vi "Teleop.vi"(10 "Match Info":T1={"Autonomous Elapsed Seconds"=0.0, "TeleOp Elapsed Seconds"=0.0, "Disabled Elapsed Seconds"=0.0, "Visited Autonomous"=FALSE, "Visited TeleOp"=FALSE, "Visited Disabled"=FALSE, "Autonomous Settings"={"Autonomous Style"=enum."Independent", "VI Refnum"=refnum}}, 11 "Call Context":T2) -> ()   [LabVIEW 2019]
doc: "This VI is called for each TeleOp packet received from the DS where the robot is not disabled. It is often used to read from the joysticks and update I/O or to update setpoints for timed control loops. It should complete and return within 20 milliseconds or it may miss DS packets."
uses:
  <vilib>/Rock Robotics/Network Tables/NT Write Numeric Array.vi
  Robot Global Data.vi
  <vilib>/Rock Robotics/Network Tables/NT Write Number.vi
  <vilib>/Rock Robotics/Network Tables/NT Write Boolean.vi
  <vilib>/Rock Robotics/Network Tables/NT Write Boolean Array.vi
  <vilib>/Rock Robotics/WPI/DriverStation/WPI_DriverStationMatch Info.ctl
  <vilib>/Rock Robotics/WPI/DriverStation/WPI_DriverStationDerivedRobotMode.ctl
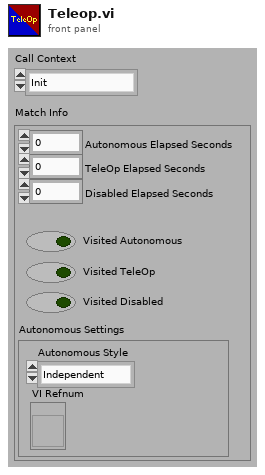
[diagram p1: front panel]
types:
  T1 = typedef "WPI_DriverStationMatch Info.ctl" = cluster{"Autonomous Elapsed Seconds":dbl, "TeleOp Elapsed Seconds":dbl, "Disabled Elapsed Seconds":dbl, "Visited Autonomous":bool, "Visited TeleOp":bool, "Visited Disabled":bool, "Autonomous Settings":cluster{"Autonomous Style":enum16{"Iterative", "Independent"}, "VI Refnum":refnum<vi>}}
  T2 = typedef "WPI_DriverStationDerivedRobotMode.ctl" = enum16{"Init", "Execute", "Stop"}
  T3 = typedef "WPI_JoystickDevRef.ctl" = cluster{"Device":T4}
  T4 = typedef "WPI_JoystickDeviceEnum.ctl" = enum16{"USB 0", "USB 1", "USB 2", "USB 3", "USB 4", "USB 5"}
  T5 = typedef "WPI_RobotDriveDevRef.ctl" = cluster{"DevStatus":errorcluster, "Motors[]":T6[], "Square Inputs":bool, "Max Output":dbl}
  T6 = typedef "WPI_MotorControlDeviceRef.ctl" = cluster{"DeviceStatus":errorcluster, "Type":T7, "PWM":cluster{"PWM Channel":T8, "DeadBand":T9}, "CAN":cluster{"Device Number":u8, "SetOutput VI Ref":variant, "GetOutput VI Ref":variant, "Enable VI Ref":variant, "Disable VI Ref":variant, "Data":variant}, "Invert":bool, "DIO PWM":cluster{"PWM \"Enable\" Channel":T8, "DIOChannel":T10, "PWM Rate":dbl}}
  T7 = typedef "WPI_MotorControlType.ctl" = enum16{"PWM", "CAN", "DIO PWM"}
  T8 = typedef "FPGA_DIOPWMChannel.ctl" = enum8{"PWM 0", "PWM 1", "PWM 2", "PWM 3", "PWM 4", "PWM 5", "PWM 6", "PWM 7", "PWM 8", "PWM 9", "PWM MXP 0", "PWM MXP 1", "PWM MXP 2", "PWM MXP 3", "PWM MXP 4", "PWM MXP 5", "PWM MXP 6", "PWM MXP 7", "PWM MXP 8", "PWM MXP 9", "Invalid"}
  T9 = typedef "WPI_PWMDeadband.ctl" = cluster{"Name":string, "maxPositivePwm":i32, "minPositivePwm":i32, "centerPwm":i32, "maxNegativePwm":i32, "minNegativePwm":i32, "angularRange":u16}
  T10 = typedef "FPGA_DIOChannel.ctl" = enum8{"DIO 0", "DIO 1", "DIO 2", "DIO 3", "DIO 4", "DIO 5", "DIO 6", "DIO 7", "DIO 8", "DIO 9", "DIO MXP 0", "DIO MXP 1", "DIO MXP 2", "DIO MXP 3", "DIO MXP 4", "DIO MXP 5", "DIO MXP 6", "DIO MXP 7", "DIO MXP 8", "DIO MXP 9", "DIO MXP 10", "DIO MXP 11", "DIO MXP 12", "DIO MXP 13", "DIO MXP 14", "DIO MXP 15", "SPI Port CS1", "SPI Port CS2", "SPI Port CS3", "SPI Port MISO", "SPI Port MOSI", "Invalid"}
  T11 = typedef "WPI_SwitchDevRef.ctl" = cluster{"DevStatus":errorcluster, "DIO Channel":T10, "CntIndex":T12, "Normally Closed":bool}
  T12 = typedef "FPGA_CounterCtrSystemIndex.ctl" = enum8{"Ctr 0", "Ctr 1", "Ctr 2", "Ctr 3", "Ctr 4", "Ctr 5", "Ctr 6", "Ctr 7", "Invalid"}
  T13 = cluster{"JoystickDevRef":T3, "RobotDriveDevRef":T5}
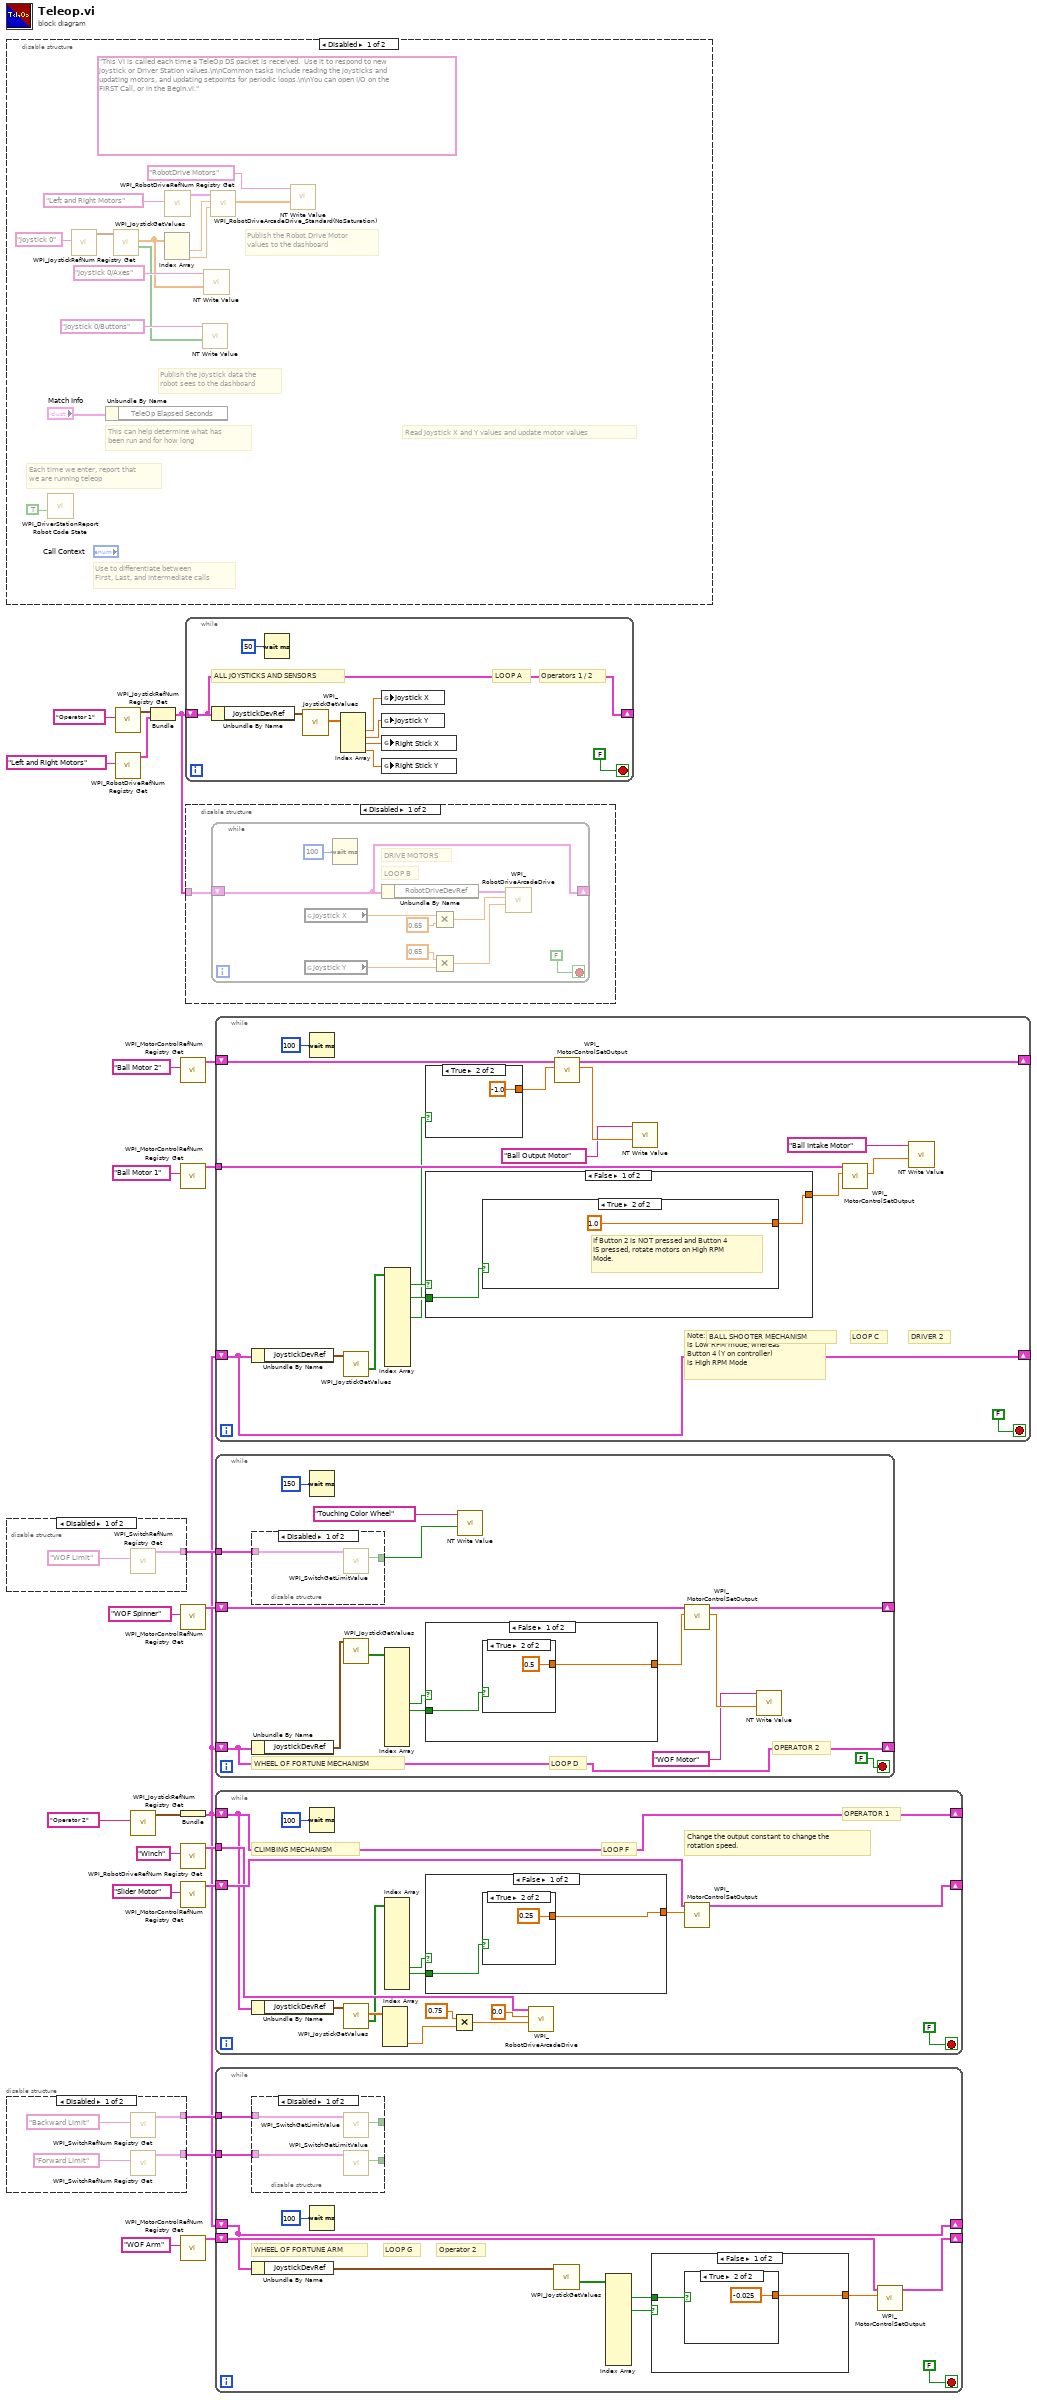
[diagram p0: block diagram]
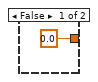
[diagram p4: hidden frame]
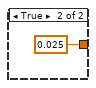
[diagram p5: hidden frame]
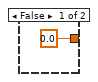
[diagram p7: hidden frame]
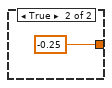
[diagram p8: hidden frame]
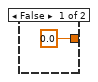
[diagram p12: hidden frame]
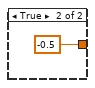
[diagram p13: hidden frame]
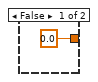
[diagram p14: hidden frame]
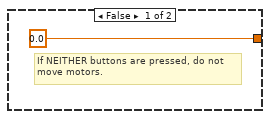
[diagram p15: hidden frame]
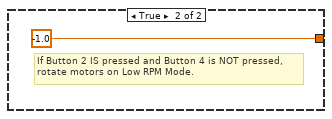
[diagram p16: hidden frame]
diagram:
  n1 = disable-structure shown="Disabled" {
    frame Disabled {
      (unwired) "This VI is called each time a TeleOp DS packet is received.  Use it to respond to new joystick or Driver Station values.\n\nCommon tasks include reading the joysticks and updating motors, and updating setpoints for periodic loops.\n\nYou can open I/O on the FIRST Call, or in the Begin.vi."
      # "Publish the Robot Drive Motor\nvalues to the dashboard"
      # "Publish the joystick data the\nrobot sees to the dashboard"
      # "Each time we enter, report that\nwe are running teleop"
      # "Use to differentiate between\nFirst, Last, and Intermediate calls"
      # "This can help determine what has\nbeen run and for how long"
      # "Read Joystick X and Y values and update motor values"
      n2 = call <vilib>:"WPI_DriverStationReport Robot Code State.vi"("TeleOp"=TRUE ("Autonomous")) -> ()  [unwired: 10 in, 1 out]
      n3 = call <vilib>:"WPI_JoystickRefNum Registry Get.vi"("refnum name"="Joystick 0") -> ("JoystickDevRef"=w32:T3)  [unwired: 1 in, 9 out]
      n4 = Unbundle By Name("Match Info") -> ()  [unwired: 1 out]
      n5 = call <vilib>:"WPI_JoystickGetValues.vi"("JoystickDevRef"=w32) -> ("Buttons"=w26:bool[], "Axes"=w27:dbl[])  [unwired: 6 in, 3 out]
      n6 = Index Array(array=w27) -> (element #1=w34:dbl, element #2=w30:dbl)  [unwired: 2 in]
      n7 = call <vilib>:"WPI_RobotDriveRefNum Registry Get.vi"("refnum name"="Left and Right Motors") -> ("RobotDriveDevRef"=w35:T5)  [unwired: 1 in, 9 out]
      n8 = call-poly <vilib>:"NT Write Value.vi"("Boolean Array"=w26, "Name"="Joystick 0/Buttons") -> ()  [unwired: 9 in, 1 out]
      n9 = call-poly <vilib>:"NT Write Value.vi"("Numeric Array"=w27, "Name"="Joystick 0/Axes") -> ()  [unwired: 9 in, 1 out]
      n10 = call <vilib>:"WPI_RobotDriveArcadeDrive_Standard(NoSaturation).vi"("Y axis value"=w30, "X axis value"=w34, "RobotDriveDevRef"=w35) -> ("Motor Values"=w25:dbl[])  [unwired: 1 in, 7 out]
      n11 = call-poly <vilib>:"NT Write Value.vi"("Numeric Array"=w25, "Name"="RobotDrive Motors") -> ()  [unwired: 9 in, 1 out]
    }
    frame Enabled {
    }
  }
  n12 = disable-structure shown="Disabled" {
    disable-tunnel: [w38 _] -> w13
    frame Disabled {
      n13 = call <vilib>:"WPI_SwitchRefNum Registry Get.vi"("refnum name"="WOF Limit") -> ("SwitchDevRef"=w38:T11)  [unwired: 9 in, 1 out]
    }
    frame Enabled {
    }
  }
  n14 = disable-structure shown="Disabled" {
    disable-tunnel: [w41 _] -> w8
    disable-tunnel: [w40 _] -> w7
    frame Disabled {
      n15 = call <vilib>:"WPI_SwitchRefNum Registry Get.vi"("refnum name"="Backward Limit") -> ("SwitchDevRef"=w40:T11)  [unwired: 9 in, 1 out]
      n16 = call <vilib>:"WPI_SwitchRefNum Registry Get.vi"("refnum name"="Forward Limit") -> ("SwitchDevRef"=w41:T11)  [unwired: 9 in, 1 out]
    }
    frame Enabled {
    }
  }
  n17 = call <vilib>:"WPI_JoystickRefNum Registry Get.vi"("refnum name"="Operator 1") -> ("JoystickDevRef"=w21:T3)  [unwired: 1 in, 9 out]
  n18 = call <vilib>:"WPI_RobotDriveRefNum Registry Get.vi"("refnum name"="Left and Right Motors") -> ("RobotDriveDevRef"=w20:T5)  [unwired: 1 in, 9 out]
  n19 = call <vilib>:"WPI_JoystickRefNum Registry Get.vi"("refnum name"="Operator 2") -> ("JoystickDevRef"=w5:T3)  [unwired: 9 in, 1 out]
  n20 = Bundle("JoystickDevRef"=w21, "RobotDriveDevRef"=w20) -> (w2:T13)  [unwired: 1 out]
  n21 = call <vilib>:"WPI_MotorControlRefNum Registry Get.vi"("refnum name"="Ball Motor 2") -> ("MotorControlDevRef"=w14:T6)  [unwired: 9 in, 1 out]
  n22 = call <vilib>:"WPI_MotorControlRefNum Registry Get.vi"("refnum name"="Ball Motor 1") -> ("MotorControlDevRef"=w18:T6)  [unwired: 9 in, 1 out]
  n23 = call <vilib>:"WPI_MotorControlRefNum Registry Get.vi"("refnum name"="WOF Spinner") -> ("MotorControlDevRef"=w16:T6)  [unwired: 9 in, 1 out]
  n24 = Bundle("JoystickDevRef"=w5) -> (w1:cluster{"JoystickDevRef":T3})  [unwired: 1 in]
  n25 = call <vilib>:"WPI_RobotDriveRefNum Registry Get.vi"("refnum name"="Winch") -> ("RobotDriveDevRef"=w4:T5)  [unwired: 9 in, 1 out]
  n26 = call <vilib>:"WPI_MotorControlRefNum Registry Get.vi"("refnum name"="Slider Motor") -> ("MotorControlDevRef"=w12:T6)  [unwired: 9 in, 1 out]
  n27 = call <vilib>:"WPI_MotorControlRefNum Registry Get.vi"("refnum name"="WOF Arm") -> ("MotorControlDevRef"=w10:T6)  [unwired: 9 in, 1 out]
  n28 = while {
    shift-right: [w51] -> _
    shift-left: w2 -> [w51]
    stop <- FALSE stop-if-true
    # "Operators 1 / 2"
    # "LOOP A"
    # "ALL JOYSTICKS AND SENSORS"
    n29 = Unbundle By Name(w51) -> ("JoystickDevRef"=w50:T3)
    n30 = Wait (ms)(milliseconds to wait=u32 50) -> ()  [unwired: 1 out]
    n31 = call <vilib>:"WPI_JoystickGetValues.vi"("JoystickDevRef"=w50) -> ("Axes"=w49:dbl[])  [unwired: 6 in, 4 out]
    n32 = Index Array(array=w49) -> (element #1=w47:dbl, element #2=w48:dbl, element #3=w45:dbl, element #4=w44:dbl)  [unwired: 4 in]
    n33 = global write "Robot Global Data.vi" "Joystick X"(w47) -> ()
    n34 = global write "Robot Global Data.vi" "Joystick Y"(w48) -> ()
    n35 = global write "Robot Global Data.vi" "Right Stick X"(w45) -> ()
    n36 = global write "Robot Global Data.vi" "Right Stick Y"(w44) -> ()
  }
  n37 = disable-structure shown="Disabled" {
    disable-tunnel: w2 -> [w53 _]
    frame Disabled {
      n38 = while {
        shift-right: [w61] -> _
        shift-left: w53 -> [w61]
        stop <- FALSE stop-if-true
        # "DRIVE MOTORS"
        # "LOOP B"
        n39 = global read "Robot Global Data.vi" "Joystick X"() -> (w58:dbl)
        n40 = global read "Robot Global Data.vi" "Joystick Y"() -> (w59:dbl)
        n41 = Wait (ms)(milliseconds to wait=u32 100) -> ()  [unwired: 1 out]
        n42 = Unbundle By Name(w61) -> ("RobotDriveDevRef"=w60:T5)
        n43 = Multiply(x=w58, y=0.65) -> (x*y=w54:dbl)
        n44 = Multiply(x=0.65, y=w59) -> (x*y=w55:dbl)
        n45 = call-poly <vilib>:"WPI_RobotDriveArcadeDrive.vi"("Y axis value"=w55, "X axis value"=w54, "RobotDriveDevRef"=w60) -> ()  [unwired: 6 in, 3 out]
      }
    }
    frame Enabled {
    }
  }
  n46 = while {
    tunnel: w18 -> [w78]
    shift-right: [w74] -> _
    shift-left: w14 -> [w75]
    shift-right: [w65] -> _
    shift-left: w1 -> [w65]
    stop <- FALSE stop-if-true
    # "DRIVER 2"
    # "LOOP C"
    # "Note: Button 2 (A on controller) \nis Low RPM mode, whereas \nButton 4 (Y on controller)\nis High RPM Mode"
    # "BALL SHOOTER MECHANISM"
    n47 = Unbundle By Name(w65) -> ("JoystickDevRef"=w64:T3)
    n48 = Wait (ms)(milliseconds to wait=u32 100) -> ()  [unwired: 1 out]
    n49 = call <vilib>:"WPI_JoystickGetValues.vi"("JoystickDevRef"=w64) -> ("Buttons"=w76:bool[])  [unwired: 6 in, 4 out]
    n50 = Index Array(array=w76) -> (element #1=w73:bool, element #3=w72:bool, element #6=w70:bool)  [unwired: 13 in, 10 out]
    n51 = case shown="True" w70 {
      tunnel: [0.0 ("Output") -1.0 ("Output")] -> w71
      frame False {
      }
      frame True {
      }
    }
    n52 = case shown="False" w73 {
      tunnel: [w84 -1.0 ("Output")] -> w77
      tunnel: w72 -> [w83 _]
      frame False {
        n53 = case shown="True" w83 {
          tunnel: [0.0 ("Output") 1.0 ("Output")] -> w84
          frame False {
            # "If NEITHER buttons are pressed, do not\nmove motors."
          }
          frame True {
            # "If Button 2 is NOT pressed and Button 4\nIS pressed, rotate motors on High RPM\nMode."
          }
        }
      }
      frame True {
        # "If Button 2 IS pressed and Button 4 is NOT pressed,\nrotate motors on Low RPM Mode."
      }
    }
    n54 = call <vilib>:"WPI_MotorControlSetOutput.vi"("Output"=w71, "MotorControlDevRef"=w75) -> ("Motor Output"=w67:dbl, "MotorControlDevRef"=w74:T6)  [unwired: 7 in, 1 out]
    n55 = call-poly <vilib>:"NT Write Value.vi"("Numeric"=w67, "Name"="Ball Output Motor") -> ()  [unwired: 9 in, 1 out]
    n56 = call <vilib>:"WPI_MotorControlSetOutput.vi"("Output"=w77, "MotorControlDevRef"=w78) -> ("Motor Output"=w69:dbl)  [unwired: 7 in, 2 out]
    n57 = call-poly <vilib>:"NT Write Value.vi"("Numeric"=w69, "Name"="Ball Intake Motor") -> ()  [unwired: 9 in, 1 out]
  }
  n58 = while {
    shift-right: [w100] -> _
    shift-left: w16 -> [w101]
    tunnel: w13 -> [w97]
    shift-right: [w89] -> _
    shift-left: w1 -> [w89]
    stop <- FALSE stop-if-true
    # "OPERATOR 2"
    # "LOOP D"
    # "WHEEL OF FORTUNE MECHANISM"
    n59 = disable-structure shown="Disabled" {
      disable-tunnel: w97 -> [w104 _]
      disable-tunnel: [w103 _] -> w95
      frame Disabled {
        n60 = call <vilib>:"WPI_SwitchGetLimitValue.vi"("SwitchDevRef"=w104) -> ("Switch Pressed"=w103:bool)  [unwired: 8 in, 2 out]
      }
      frame Enabled {
      }
    }
    n61 = Unbundle By Name(w89) -> ("JoystickDevRef"=w88:T3)
    n62 = Wait (ms)(milliseconds to wait=u32 150) -> ()  [unwired: 1 out]
    n63 = call <vilib>:"WPI_JoystickGetValues.vi"("JoystickDevRef"=w88) -> ("Buttons"=w94:bool[])  [unwired: 6 in, 4 out]
    n64 = Index Array(array=w94) -> (element #7=w93:bool, element #8=w92:bool)  [unwired: 13 in, 11 out]
    n65 = case shown="False" w93 {
      tunnel: [w106 -0.5 ("Output")] -> w99
      tunnel: w92 -> [w105 _]
      frame False {
        n66 = case shown="True" w105 {
          tunnel: [0.0 ("Output") 0.5 ("Output")] -> w106
          frame False {
          }
          frame True {
          }
        }
      }
      frame True {
      }
    }
    n67 = call-poly <vilib>:"NT Write Value.vi"("Boolean"=w95, "Name"="Touching Color Wheel") -> ()  [unwired: 9 in, 1 out]
    n68 = call <vilib>:"WPI_MotorControlSetOutput.vi"("Output"=w99, "MotorControlDevRef"=w101) -> ("Motor Output"=w91:dbl, "MotorControlDevRef"=w100:T6)  [unwired: 7 in, 1 out]
    n69 = call-poly <vilib>:"NT Write Value.vi"("Numeric"=w91, "Name"="WOF Motor") -> ()  [unwired: 9 in, 1 out]
  }
  n70 = while {
    shift-right: [w110] -> _
    shift-left: w12 -> [w125]
    tunnel: w4 -> [w120]
    shift-right: [w112] -> _
    shift-left: w1 -> [w112]
    stop <- FALSE stop-if-true
    # "Change the output constant to change the\nrotation speed."
    # "OPERATOR 1"
    # "LOOP F"
    # "CLIMBING MECHANISM"
    n71 = Unbundle By Name(w112) -> ("JoystickDevRef"=w111:T3)
    n72 = Wait (ms)(milliseconds to wait=u32 100) -> ()  [unwired: 1 out]
    n73 = call <vilib>:"WPI_JoystickGetValues.vi"("JoystickDevRef"=w111) -> ("Buttons"=w115:bool[], "Axes"=w121:dbl[])  [unwired: 6 in, 3 out]
    n74 = Index Array(array=w121) -> (element #4=w117:dbl)  [unwired: 4 in, 3 out]
    n75 = Index Array(array=w115) -> (element #9=w114:bool, element #10=w113:bool)  [unwired: 12 in, 10 out]
    n76 = case shown="False" w114 {
      tunnel: [w127 -0.25 ("Output")] -> w123
      tunnel: w113 -> [w126 _]
      frame False {
        n77 = case shown="True" w126 {
          tunnel: [0.0 ("Output") 0.25 ("Output")] -> w127
          frame False {
          }
          frame True {
          }
        }
      }
      frame True {
      }
    }
    n78 = Multiply(x=0.75, y=w117) -> (x*y=w118:dbl)
    n79 = call-poly <vilib>:"WPI_RobotDriveArcadeDrive.vi"("Y axis value"=w118, "X axis value"=0.0, "RobotDriveDevRef"=w120) -> ()  [unwired: 6 in, 3 out]
    n80 = call <vilib>:"WPI_MotorControlSetOutput.vi"("Output"=w123, "MotorControlDevRef"=w125) -> ("MotorControlDevRef"=w110:T6)  [unwired: 7 in, 2 out]
  }
  n81 = while {
    shift-right: [w141] -> _
    shift-left: w10 -> [w140]
    tunnel: w8 -> [w138]
    tunnel: w7 -> [w137]
    shift-right: [w132] -> _
    shift-left: w1 -> [w132]
    stop <- FALSE stop-if-true
    # "LOOP G"
    # "Operator 2"
    # "WHEEL OF FORTUNE ARM"
    n82 = disable-structure shown="Disabled" {
      disable-tunnel: w138 -> [w151 _]
      disable-tunnel: w137 -> [w150 _]
      disable-tunnel: [w149 _] -> _
      disable-tunnel: [w148 _] -> _
      frame Disabled {
        n83 = call <vilib>:"WPI_SwitchGetLimitValue.vi"("SwitchDevRef"=w150) -> ("Switch Pressed"=w148:bool)  [unwired: 8 in, 2 out]
        n84 = call <vilib>:"WPI_SwitchGetLimitValue.vi"("SwitchDevRef"=w151) -> ("Switch Pressed"=w149:bool)  [unwired: 8 in, 2 out]
      }
      frame Enabled {
      }
    }
    n85 = Unbundle By Name(w132) -> ("JoystickDevRef"=w131:T3)
    n86 = Wait (ms)(milliseconds to wait=u32 100) -> ()  [unwired: 1 out]
    n87 = call <vilib>:"WPI_JoystickGetValues.vi"("JoystickDevRef"=w131) -> ("Buttons"=w139:bool[])  [unwired: 6 in, 4 out]
    n88 = Index Array(array=w139) -> (element #2=w134:bool, element #4=w136:bool)  [unwired: 12 in, 10 out]
    n89 = case shown="False" w136 {
      tunnel: [w143 0.025 ("Output")] -> w135
      tunnel: w134 -> [w144 _]
      frame False {
        n90 = case shown="True" w144 {
          tunnel: [0.0 ("Output") -0.025 ("Output")] -> w143
          frame False {
          }
          frame True {
          }
        }
      }
      frame True {
      }
    }
    n91 = call <vilib>:"WPI_MotorControlSetOutput.vi"("Output"=w135, "MotorControlDevRef"=w140) -> ("MotorControlDevRef"=w141:T6)  [unwired: 7 in, 2 out]
  }
